vi "Config Sample Switch.vi"(8 "error in":errorcluster, 10 "Sample Switch (1)":i32=1 min=1 max=64, 11 "VISA resource name":refnum<visa-resource-name>) -> (0 "error out":errorcluster, 3 "VISA resource name out":refnum<visa-resource-name>)   [LabVIEW 2017, in "Andeen-Hagerling 2700.lvlib"]
doc: "This VI selects which external unknown sample to measure. Operates only in conjunction with the sample switch port."
uses:
  Andeen-Hagerling 2700.lvlib
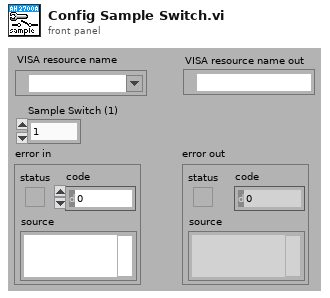
[diagram p1: front panel]
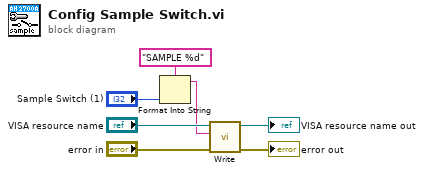
[diagram p0: block diagram]
diagram:
  n1 = Format Into String(format string="SAMPLE %d", "Sample Switch (1)") -> (resulting string=w4:string)  [unwired: 2 in, 1 out]
  n2 = call "Write.vi"("error in"="error in", "command"=w4, "VISA resource name"="VISA resource name") -> ("error out"=→"error out":errorcluster, "VISA resource name out"=→"VISA resource name out":refnum<visa-resource-name>)  [unwired: 7 in]
